vi "battery-reader-dialog.vi"() -> ()   [LabVIEW 2025]
uses:
  <vilib>/addons/_JKI Toolkits/State Machine/_JKI_lib_State_Machine.llb/Select State(s)_err__jki_lib_state_machine.vi
  <vilib>/addons/_JKI Toolkits/State Machine/_JKI_lib_State_Machine.llb/Periodic Trigger__ogtk__JKI-SM__jki_lib_state_machine.vi
panel:
  in  "Exit 2":bool
  in  "Exit":bool
  in  "Select":bool
  in  "Image selection":enum32{"Camera", "File input"}(tab)
  in  "Pict Ring":u16(ring)
  out "error out":errorcluster
  in  "error in":errorcluster
  in  "Camera ID":u8
  # "1. Select the camera ID and read the image."
  # "2. Use camera input, or select one of the predefined templates."
  # "3."
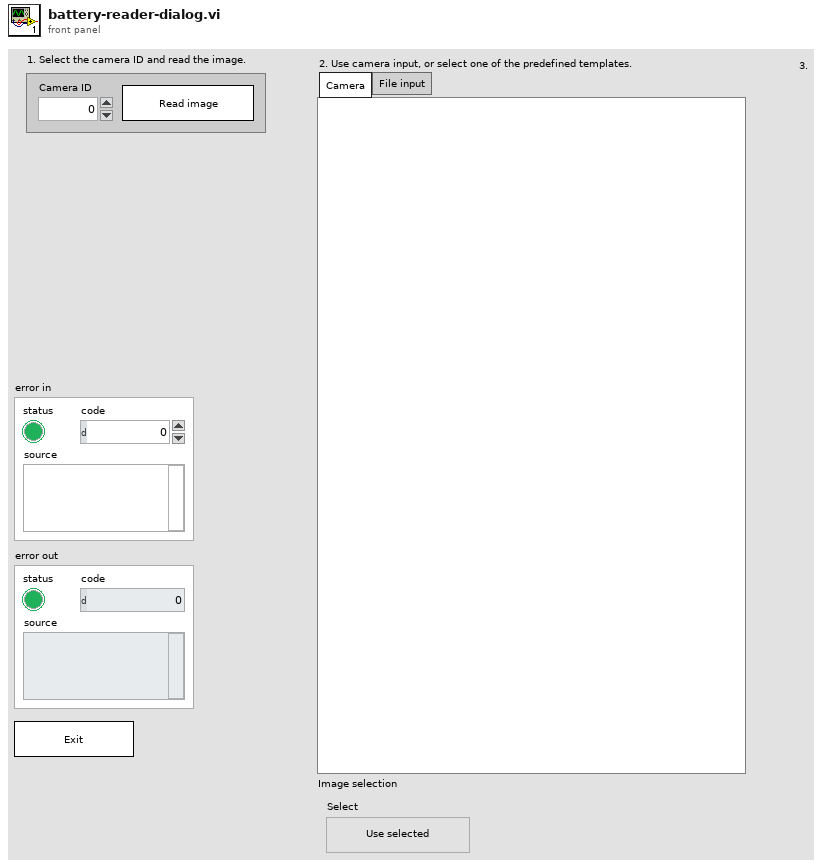
[diagram p1: front panel]
types:
  T1 = enum32{"Invalid", "Standard", "Closed", "Hidden", "Minimized", "Maximized"}
  T2 = enum32{"invalid app kind", "Development System", "Run Time System", "Student Edition", "Embedded LabVIEW", "Evaluation", "Custom"}
  T3 = cluster{"Core":cluster{"Current VI Reference":refnum<vi>, "Close Panel on Exit?":bool}, "Your Boolean data":bool, "Your string data":string}
  T4 = cluster{"Current VI Reference":refnum<vi>, "Close Panel on Exit?":bool}
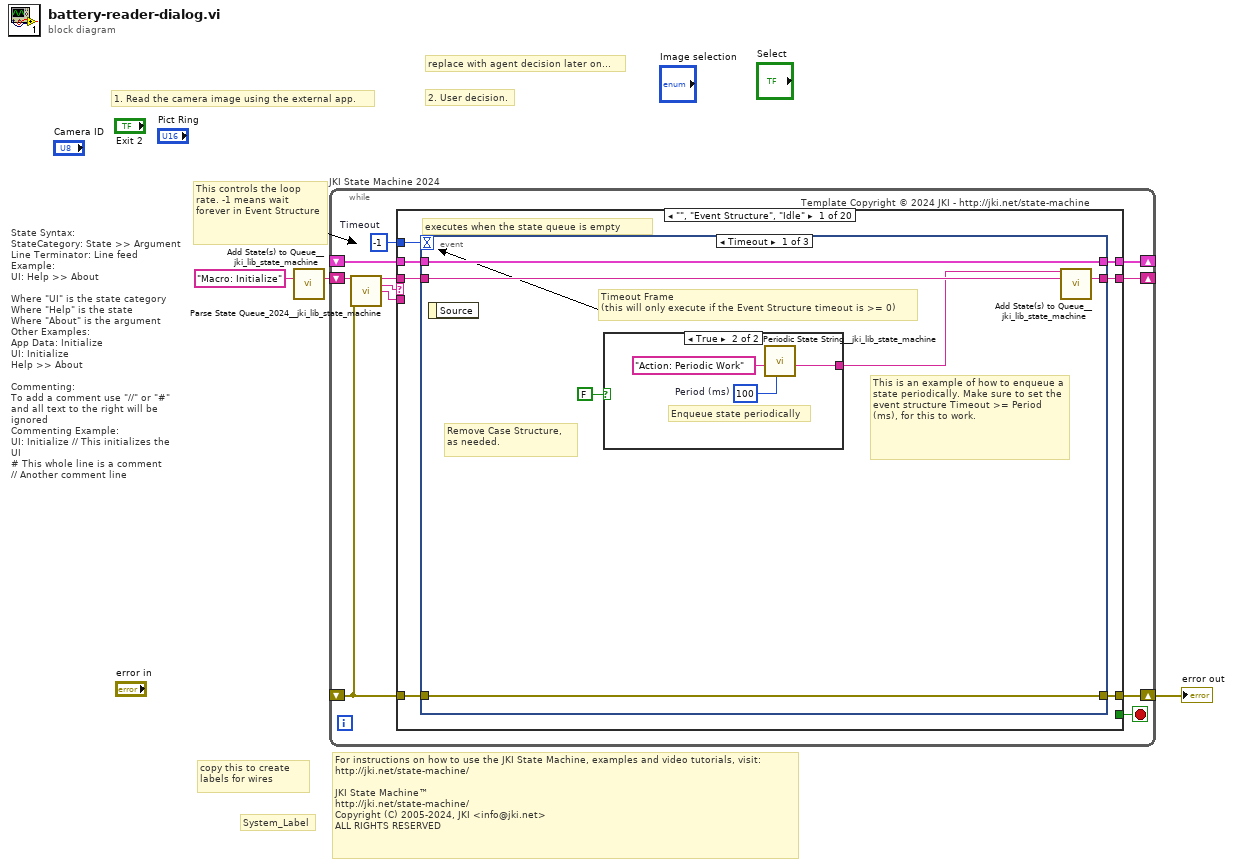
[diagram p0: block diagram]
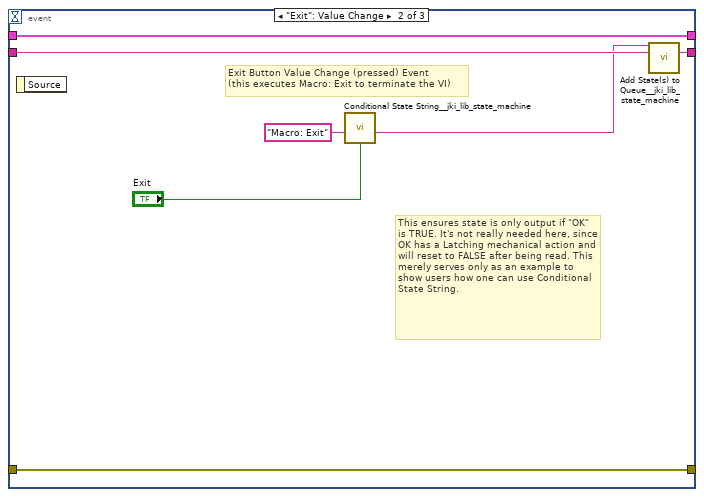
[diagram p3: hidden frame]
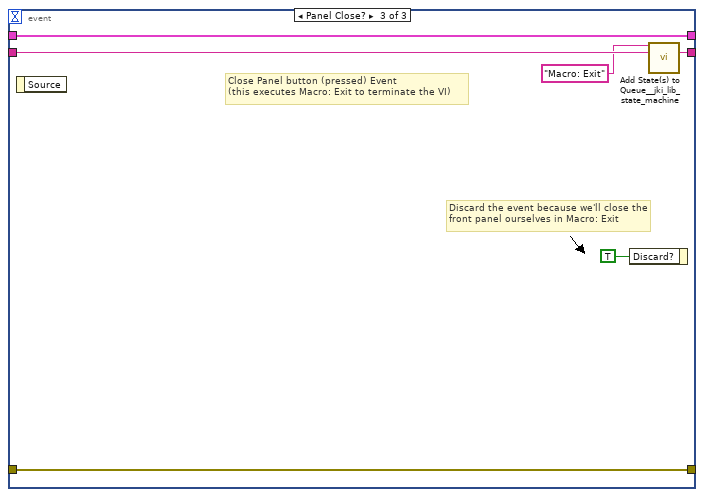
[diagram p4: hidden frame]
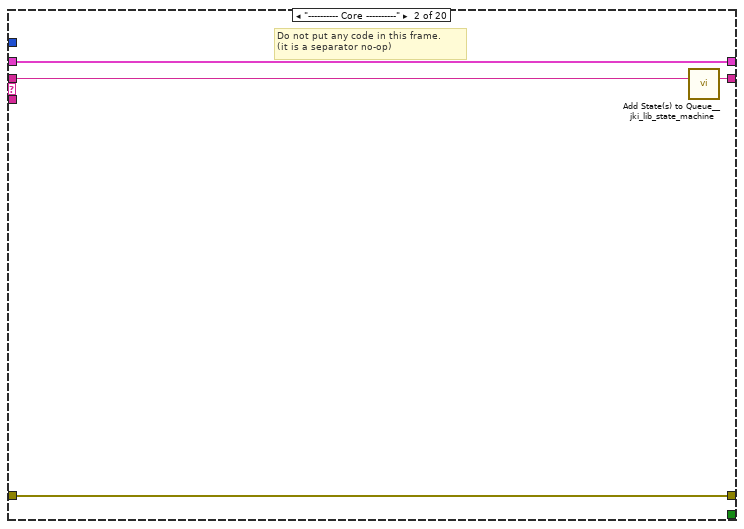
[diagram p5: hidden frame]
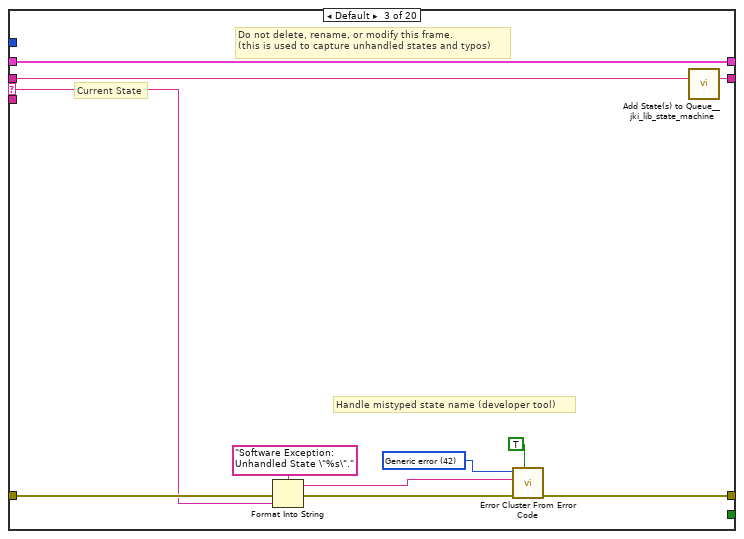
[diagram p6: hidden frame]
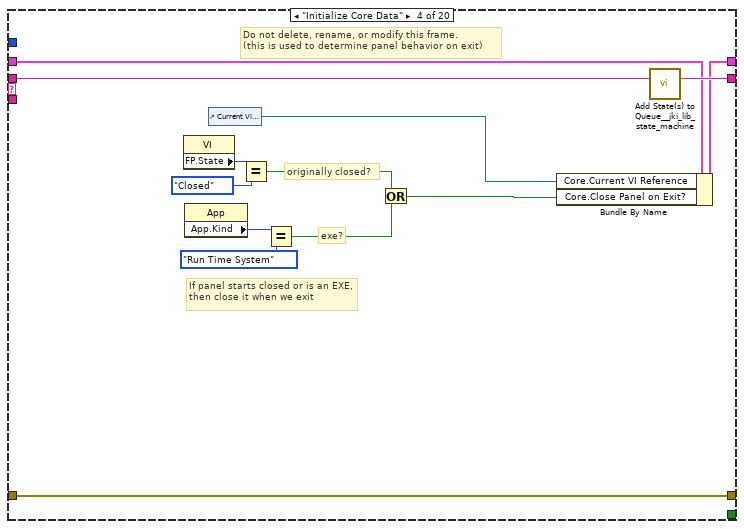
[diagram p7: hidden frame]
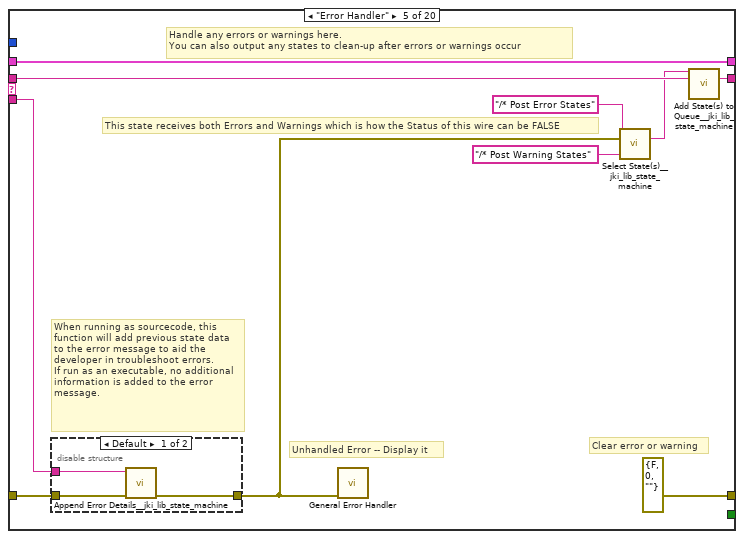
[diagram p8: hidden frame]
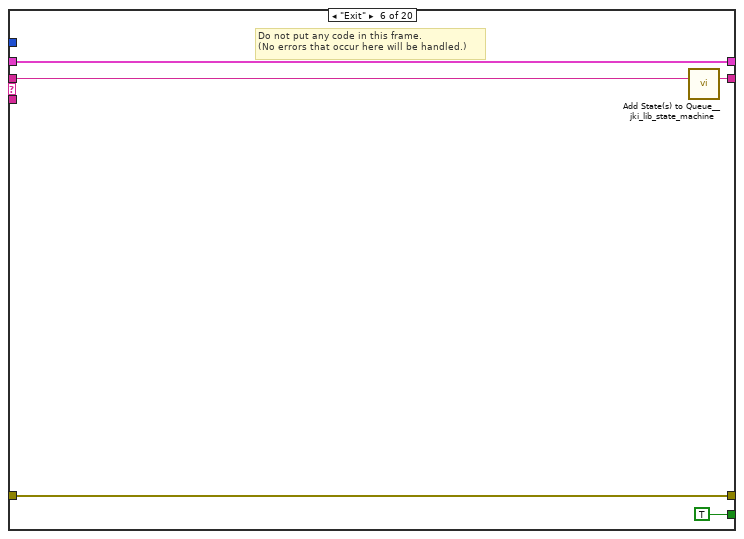
[diagram p10: hidden frame]
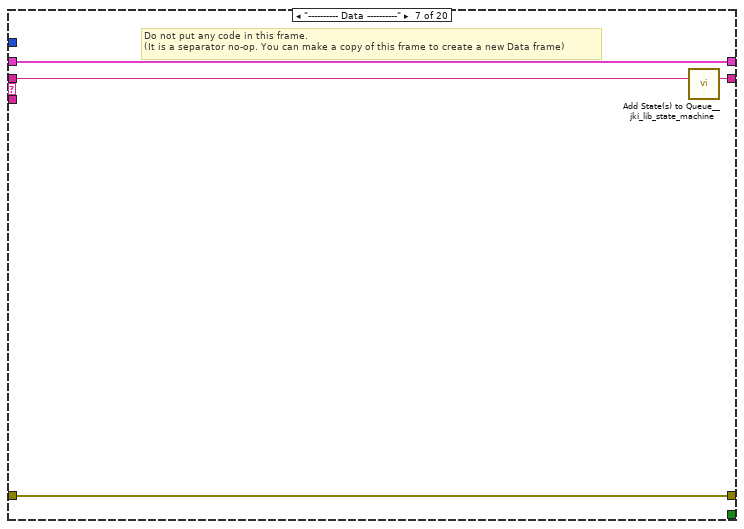
[diagram p11: hidden frame]
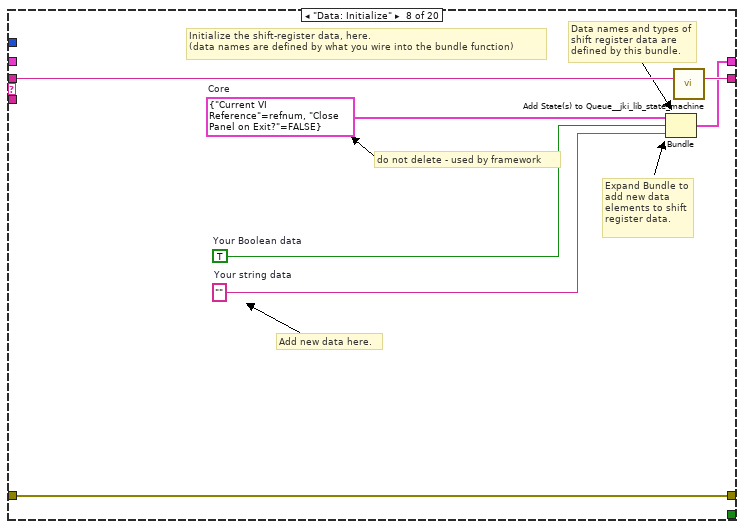
[diagram p12: hidden frame]
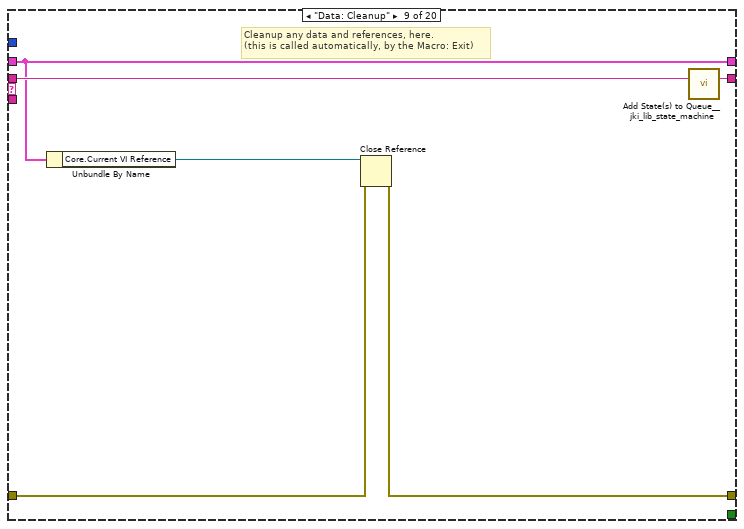
[diagram p13: hidden frame]
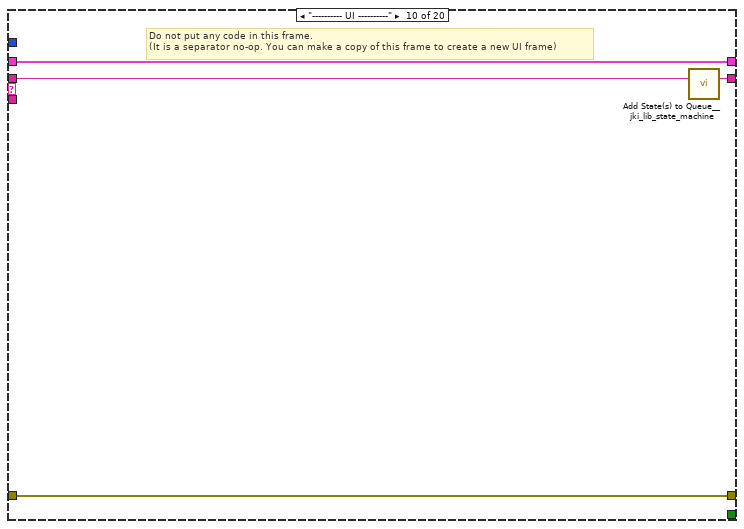
[diagram p14: hidden frame]
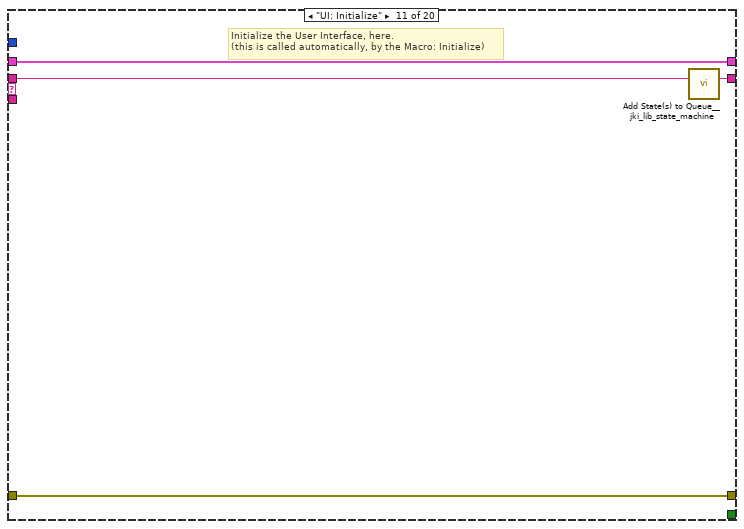
[diagram p15: hidden frame]
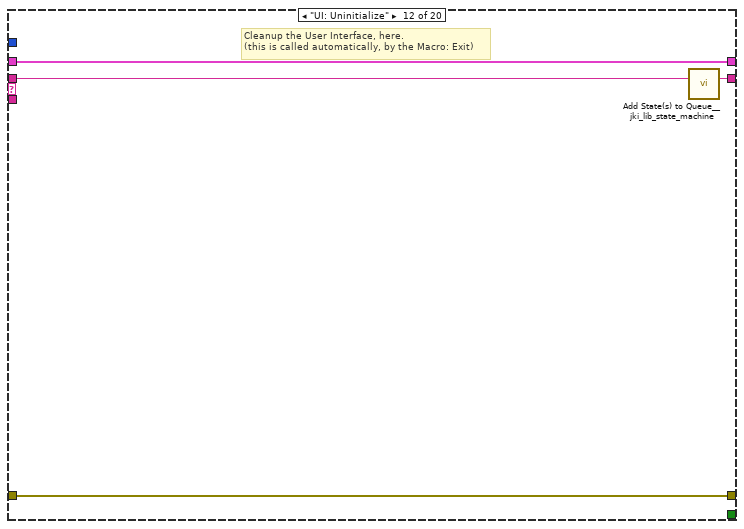
[diagram p16: hidden frame]
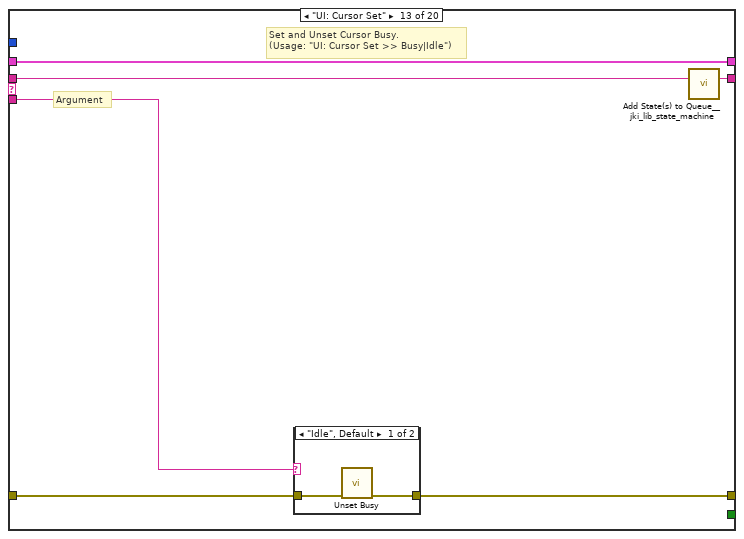
[diagram p17: hidden frame]
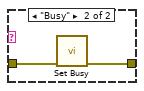
[diagram p18: hidden frame]
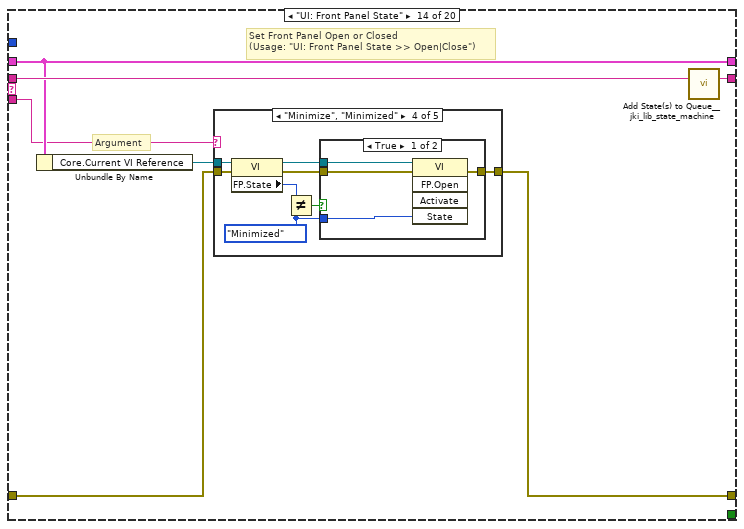
[diagram p19: hidden frame]
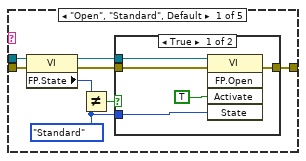
[diagram p20: hidden frame]
diagram:
  # "For instructions on how to use the JKI State Machine, examples and video tutorials, visit:\nhttp://jki.net/state-machine/\n\nJKI State Machine™\nhttp://jki.net/state-machine/\nCopyright (C) 2005-2024, JKI <info@jki.net>\nALL RIGHTS RESERVED"
  # "State Syntax:\nStateCategory: State >> Argument\nLine Terminator: Line feed\nExample:\nUI: Help >> About\n\nWhere \"UI\" is the state category\nWhere \"Help\" is the state\nWhere \"About\" is the argument\nOther Examples:\nApp Data: Initialize\nUI: Initialize\nHelp >> About\n\nCommenting:\nTo add a comment use \"//\" or \"#\" and all text to the right will be ignored\nCommenting Example:\nUI: Initialize // This initializes the UI\n# This whole line is a comment\n// Another comment line"
  # "copy this to create labels for wires"
  # "This controls the loop rate. -1 means wait forever in Event Structure"
  # "System_Label"
  # "replace with agent decision later on..."
  # "2. User decision."
  # "1. Read the camera image using the external app."
  n1 = call <vilib>:"Add State(s) to Queue__jki_lib_state_machine.vi"("State(s) in (\"\")"="Macro: Initialize") -> ("States Out"=w3:string)  [unwired: 14 in]
  n2 = while "JKI State Machine 2024" {
    shift-right: [w7] -> _
    shift-left: _ -> [w6]
    shift-right: [w10] -> w1
    shift-left: _ -> [w4]
    shift-right: [w9] -> _
    shift-left: w3 -> [w11]
    stop <- w8 stop-if-true
    w5 = -1  # Timeout
    # "Template Copyright © 2024 JKI - http://jki.net/state-machine"
    n3 = call <vilib>:"Parse State Queue_2024__jki_lib_state_machine.vi"("State Queue"=w11, "Error In (no error)"=w4) -> ("Remaining States"=w13:string, "Current State"=w14:string, "Arguments"=w12:string)  [unwired: 11 in]
    n4 = case shown="\"\", \"Event Structure\", \"Idle\"" w14 {
      selector: w14 -> [_ _ w48 _ _ _ _ _ _ _ _ _ _ _ _ _ _ _ _ _]
      tunnel: w13 -> [w21 w47 w52 w71 w81 w90 w94 w101 w107 w111 w115 w119 w125 w136 w205 w210 w219 w223 w227 w231]
      tunnel: w12 -> [_ _ _ _ w76 _ _ _ _ _ _ _ w120 w130 _ _ _ _ _ _]
      tunnel: w6 -> [w19 w44 w50 w64 w78 w88 w91 _ w102 w108 w113 w117 w123 w132 w202 w207 w217 w220 w224 w228]
      tunnel: [w18 w45 w54 w68 errorcluster {"status"=FALSE, "code"=0, "source"=""} ("error out") w87 w92 w98 w103 w109 w112 w116 w121 w133 w203 w208 w214 w221 w225 w229] -> w10
      tunnel: w4 -> [w15 w45 w53 w68 w77 w87 w92 w98 w104 w109 w112 w116 w122 w134 w203 w208 w214 w221 w225 w229]
      tunnel: [w20 w46 w51 w70 w80 w89 w93 w100 w106 w110 w114 w118 w124 w135 w204 w209 w218 w222 w226 w230] -> w9
      tunnel: [_ _ _ _ _ TRUE _ _ _ _ _ _ _ _ _ _ _ _ _ _] -> w8
      tunnel: [w17 w44 w50 w69 w78 w88 w91 w99 w102 w108 w113 w117 w123 w132 w202 w207 w217 w220 w224 w228] -> w7
      tunnel: w5 -> [w16 _ _ _ _ _ _ _ _ _ _ _ _ _ _ _ _ _ _ _]
      frame "", "Event Structure", "Idle" {
        # "executes when the state queue is empty"
        n5 = event shown="[0] Timeout" {
          selector: _ -> [_ _ _]
          dyn-events: _ -> [_ _ _]
          timeout: w16 -> [_ _ _]
          tunnel: w21 -> [w27 w37 w43]
          tunnel: [w26 w36 w42] -> w20
          tunnel: w19 -> [w24 w34 w40]
          tunnel: [w25 w35 w41] -> w18
          tunnel: w15 -> [w25 w35 w41]
          tunnel: [w24 w34 w40] -> w17
          event Timeout {
            # "Remove Case Structure, as needed."
            # "This is an example of how to enqueue a state periodically. Make sure to set the event structure Timeout >= Period (ms), for this to work."
            # "Timeout Frame\n(this will only execute if the Event Structure timeout is >= 0)"
            n6 = event-data() -> ()  [unwired: 1 in, 1 out]
            n7 = case shown="True" FALSE {
              tunnel: [_ w30] -> w23
              frame False {
              }
              frame True {
                w28 = u32 100  # Period (ms)
                # "Enqueue state periodically"
                n8 = call <vilib>:"Periodic State String__jki_lib_state_machine.vi"("Period (ms)"=w28, "State"="Action: Periodic Work") -> ("State Out"=w30:string)  [unwired: 9 in]
              }
            }
            n9 = call <vilib>:"Add State(s) to Queue__jki_lib_state_machine.vi"("State(s) in Front (\"\")"=w23, "State(s) in (\"\")"=w27) -> ("States Out"=w26:string)  [unwired: 13 in]
          }
          event "Exit": Value Change {
            # "This ensures state is only output if \"OK\" is TRUE. It's not really needed here, since OK has a Latching mechanical action and will reset to FALSE after being read. This merely serves only as an example to show users how one can use Conditional State String."
            # "Exit Button Value Change (pressed) Event\n(this executes Macro: Exit to terminate the VI)"
            n10 = event-data() -> ()  [unwired: 1 in, 1 out]
            n11 = call <vilib>:"Conditional State String__jki_lib_state_machine.vi"("Do State(s)?"="Exit", "State"="Macro: Exit") -> ("State Out"=w31:string)  [unwired: 7 in]
            n12 = call <vilib>:"Add State(s) to Queue__jki_lib_state_machine.vi"("State(s) in Front (\"\")"=w31, "State(s) in (\"\")"=w37) -> ("States Out"=w36:string)  [unwired: 13 in]
          }
          event Panel Close? {
            # "Discard the event because we'll close the front panel ourselves in Macro: Exit"
            # "Close Panel button (pressed) Event\n(this executes Macro: Exit to terminate the VI)"
            n13 = event-data() -> ()  [unwired: 1 in, 1 out]
            n14 = event-data("Discard?"=TRUE) -> ()  [unwired: 1 in, 1 out]
            n15 = call <vilib>:"Add State(s) to Queue__jki_lib_state_machine.vi"("State(s) in Front (\"\")"="Macro: Exit", "State(s) in (\"\")"=w43) -> ("States Out"=w42:string)  [unwired: 13 in]
          }
        }
      }
      frame "---------- Core ----------" {
        # "Do not put any code in this frame.\n(it is a separator no-op)"
        n16 = call <vilib>:"Add State(s) to Queue__jki_lib_state_machine.vi"("State(s) in (\"\")"=w47) -> ("States Out"=w46:string)  [unwired: 14 in]
      }
      frame Default {
        w57 = 42 items=["No error", "Argument error", "Memory is full", "Out of zone", "End of file", "File already open", "Generic file I/O error", "File not found", "File permission error", "Disk is full", "Duplicate path", "Too many files open", "System feature not enabled", "Resource file not found", "Cannot add resource", "Resource not found", "Image not found", "Image memory error", "Pen does not exist", "Config type invalid", "Config token not found", "Config parse error", "Config memory error", "Bad external code format", "Bad external code offset", "External code not present", "Null window", "Destroy window error", "Null menu", "Print aborted", "Bad print record", "Print driver error", "Windows error during printing", "Memory error during printing", "Print dialog error", "Generic print error", "Invalid device refnum", "Device not found", "Device parameter error", "Device unit error", "Cannot open device", "Device call aborted", "Generic error", "Cancelled by user", "Object ID too low", "Object ID too high", "Object not in heap", "Unknown heap", "Unknown object (invalid DefProc)", "Unknown object (DefProc not in table)", "Message out of range", "Invalid (null) method", "Unknown message", "Manager call not supported", "Bad address", "Network operation in progress", "Network operation timed out", "Connection is busy", "Network attribute not supported", "Network error", "Address in use", "System out of memory", "Connection aborted", "Connection refused", "Not connected", "Already connected", "Connection closed", "Initialization error (interapplication manager)", "Bad occurrence", "Wait on unbound occurrence handler", "Occurrence queue overflow", "Datalog type conflict", "Unused", "Unrecognized type (interapplication manager)", "Memory corrupt", "Failed to make temporary DLL", "Old CIN version", "Drag socket not found", "Failed to load drop-object", "Failed to register OLE object", "Failed to release OLE object", "Format specifier type mismatch", "Unknown format specifier", "Too few format specifiers", "Too many format specifiers", "Scan failed", "Newer CIN version", "Error converting to variant", "Runtime menu error", "Password tampered", "Variant attribute not found", "Incompatible variant data type", "Event data is not available", "Event Store is not present", "Occurrence is not found", "Event Queue is not created", "Event info is not available", "Refnum passed is NULL", "Error retrieving Class GUID", "Error retrieving CoClass GUID", "Error retrieving TypeLib GUID.", "Bad built application magic bytes.", "Specific driver is different from the specific driver associated with the Logical Name.", "There is no session opened to the class driver.", "Max Error", "MAX - Error with config objects", "MAX - Error loading configuration", "MAX - Group not supported"]
        # "Current State"
        # "Do not delete, rename, or modify this frame.\n(this is used to capture unhandled states and typos)"
        # "Handle mistyped state name (developer tool)"
        n17 = Format Into String(format string="Software Exception: Unhandled State \"%s\"." ("message"), error in=w53, w48) -> (resulting string=w56:string, error out=w55:errorcluster)  [unwired: 1 in]
        n18 = call <vilib>:"Error Cluster From Error Code.vi"("show call chain? (False)"=TRUE, "error in (no error)"=w55, "error message (\"\")"=w56, "error code (0)"=w57) -> ("error out"=w54:errorcluster)  [unwired: 5 in]
        n19 = call <vilib>:"Add State(s) to Queue__jki_lib_state_machine.vi"("State(s) in (\"\")"=w52) -> ("States Out"=w51:string)  [unwired: 14 in]
      }
      frame "Initialize Core Data" {
        # "Do not delete, rename, or modify this frame.\n(this is used to determine panel behavior on exit)"
        # "originally closed?"
        # "exe?"
        # "If panel starts closed or is an EXE, then close it when we exit"
        n20 = property class="VI"() -> ("FP.State"=w61:T1)  [unwired: 2 in, 2 out]
        n21 = property class="App"() -> ("App.Kind"=w67:T2)  [unwired: 2 in, 2 out]
        n22 = control-ref of="Current VI Reference"() -> (w62:refnum<vi>)
        n23 = Equal?(x=w61, y=T1."Closed" ("Front Panel Window:State")) -> (x = y?=w59:bool)
        n24 = Equal?(x=w67, y=T2."Run Time System" ("Application:Kind")) -> (x = y?=w65:bool)
        n25 = Or(x=w59, y=w65) -> (x .or. y?=w63:bool)
        n26 = Bundle By Name(cluster=w64, "Core.Current VI Reference"=w62, "Core.Close Panel on Exit?"=w63) -> (w69:T3)
        n27 = call <vilib>:"Add State(s) to Queue__jki_lib_state_machine.vi"("State(s) in (\"\")"=w71) -> ("States Out"=w70:string)  [unwired: 14 in]
      }
      frame "Error Handler" {
        # "When running as sourcecode, this function will add previous state data to the error message to aid the developer in troubleshoot errors.\nIf run as an executable, no additional information is added to the error message."
        # "This state receives both Errors and Warnings which is how the Status of this wire can be FALSE"
        # "Unhandled Error -- Display it"
        # "Handle any errors or warnings here.\nYou can also output any states to clean-up after errors or warnings occur"
        # "Clear error or warning"
        n28 = disable-structure shown="Default" {
          disable-tunnel: w77 -> [w84 w85]
          disable-tunnel: w76 -> [w83 _]
          disable-tunnel: [w82 w85] -> w75
          frame condition #0 (active) {
            n29 = call <vilib>:"Append Error Details__jki_lib_state_machine.vi"("error in (no error)"=w84, "Previous State and Argument(s)"=w83) -> ("error out"=w82:errorcluster)  [unwired: 9 in]
          }
          frame condition #1 {
          }
        }
        n30 = call <vilib>:"General Error Handler.vi"("error in (no error)"=w75) -> ()  [unwired: 10 in, 5 out]
        n31 = call-poly <vilib>:"Select State(s)__jki_lib_state_machine.vi"("State(s) if True (\"\")"="/* Post Error States", "Select"=w75, "State(s) if False (\"\")"="/* Post Warning States") -> ("States Out"=w73:string)  [unwired: 12 in]
        n32 = call <vilib>:"Add State(s) to Queue__jki_lib_state_machine.vi"("State(s) in Front (\"\")"=w73, "State(s) in (\"\")"=w81) -> ("States Out"=w80:string)  [unwired: 13 in]
      }
      frame "Exit" {
        # "Do not put any code in this frame.\n(No errors that occur here will be handled.)"
        n33 = call <vilib>:"Add State(s) to Queue__jki_lib_state_machine.vi"("State(s) in (\"\")"=w90) -> ("States Out"=w89:string)  [unwired: 14 in]
      }
      frame "---------- Data ----------" {
        # "Do not put any code in this frame.\n(It is a separator no-op. You can make a copy of this frame to create a new Data frame)"
        n34 = call <vilib>:"Add State(s) to Queue__jki_lib_state_machine.vi"("State(s) in (\"\")"=w94) -> ("States Out"=w93:string)  [unwired: 14 in]
      }
      frame "Data: Initialize" {
        w95 = T4 {"Current VI Reference"=refnum, "Close Panel on Exit?"=FALSE}  # Core
        w97 = TRUE  # Your Boolean data
        w96 = ""  # Your string data
        # "do not delete - used by framework"
        # "Expand Bundle to add new data elements to shift register data."
        # "Add new data here."
        # "Data names and types of shift register data are defined by this bundle."
        # "Initialize the shift-register data, here.\n(data names are defined by what you wire into the bundle function)"
        n35 = Bundle("Core"=w95, "Your Boolean data"=w97, "Your string data"=w96) -> (w99:T3)  [unwired: 1 in]
        n36 = call <vilib>:"Add State(s) to Queue__jki_lib_state_machine.vi"("State(s) in (\"\")"=w101) -> ("States Out"=w100:string)  [unwired: 14 in]
      }
      frame "Data: Cleanup" {
        # "Cleanup any data and references, here.\n(this is called automatically, by the Macro: Exit)"
        n37 = Unbundle By Name(w102) -> ("Core.Current VI Reference"=w105:refnum<vi>)
        n38 = Close Reference(reference=w105, error in (no error)=w104) -> (error out=w103:errorcluster)
        n39 = call <vilib>:"Add State(s) to Queue__jki_lib_state_machine.vi"("State(s) in (\"\")"=w107) -> ("States Out"=w106:string)  [unwired: 14 in]
      }
      frame "---------- UI ----------" {
        # "Do not put any code in this frame.\n(It is a separator no-op. You can make a copy of this frame to create a new UI frame)"
        n40 = call <vilib>:"Add State(s) to Queue__jki_lib_state_machine.vi"("State(s) in (\"\")"=w111) -> ("States Out"=w110:string)  [unwired: 14 in]
      }
      frame "UI: Initialize" {
        # "Initialize the User Interface, here.\n(this is called automatically, by the Macro: Initialize)"
        n41 = call <vilib>:"Add State(s) to Queue__jki_lib_state_machine.vi"("State(s) in (\"\")"=w115) -> ("States Out"=w114:string)  [unwired: 14 in]
      }
      frame "UI: Uninitialize" {
        # "Cleanup the User Interface, here.\n(this is called automatically, by the Macro: Exit)"
        n42 = call <vilib>:"Add State(s) to Queue__jki_lib_state_machine.vi"("State(s) in (\"\")"=w119) -> ("States Out"=w118:string)  [unwired: 14 in]
      }
      frame "UI: Cursor Set" {
        # "Argument"
        # "Set and Unset Cursor Busy.\n(Usage: \"UI: Cursor Set >> Busy|Idle\")"
        n43 = case shown="\"Idle\", Default" w120 {
          tunnel: w122 -> [w127 w129]
          tunnel: [w126 w128] -> w121
          frame "Idle", Default {
            n44 = call <vilib>:"Unset Busy.vi"("error in (no error)"=w127) -> ("error out"=w126:errorcluster)  [unwired: 10 in]
          }
          frame "Busy" {
            n45 = call <vilib>:"Set Busy.vi"("error in (no error)"=w129) -> ("error out"=w128:errorcluster)  [unwired: 9 in, 1 out]
          }
        }
        n46 = call <vilib>:"Add State(s) to Queue__jki_lib_state_machine.vi"("State(s) in (\"\")"=w125) -> ("States Out"=w124:string)  [unwired: 14 in]
      }
      frame "UI: Front Panel State" {
        # "Argument"
        # "Set Front Panel Open or Closed\n(Usage: \"UI: Front Panel State >> Open|Close\")"
        n47 = Unbundle By Name(w132) -> ("Core.Current VI Reference"=w131:refnum<vi>)
        n48 = case shown="\"Minimize\", \"Minimized\"" w130 {
          tunnel: w134 -> [w142 w157 w168 w181 w194]
          tunnel: [w144 w158 w170 w183 w196] -> w133
          tunnel: w131 -> [w143 w155 w169 w182 w195]
          frame "Open", "Standard", Default {
            w137 = T1."Standard" ("State")
            n49 = property class="VI"(reference=w143, error in=w142) -> (reference out=w140:refnum<vi>, error out=w141:errorcluster, "FP.State"=w139:T1)
            n50 = Not Equal?(x=w139, y=w137) -> (x != y?=w138:bool)
            n51 = case shown="True" w138 {
              tunnel: [w148 w150] -> w144
              tunnel: w141 -> [w147 w150]
              tunnel: w140 -> [w146 _]
              tunnel: w137 -> [w145 _]
              frame True {
                n52 = invoke class="VI" method="FP.Open"(reference=w146, error in=w147, "Activate"=TRUE, "State"=w145) -> (error out=w148:errorcluster)  [unwired: 1 in, 4 out]
              }
              frame False {
              }
            }
          }
          frame "Close", "Closed" {
            n53 = property class="VI"(reference=w155, error in=w157) -> (reference out=w154:refnum<vi>, error out=w156:errorcluster, "FP.State"=w152:T1)
            n54 = Not Equal?(x=w152, y=T1."Closed" ("Front Panel Window:State")) -> (x != y?=w151:bool)
            n55 = case shown="True" w151 {
              tunnel: [w159 w162] -> w158
              tunnel: w156 -> [w159 w161]
              tunnel: w154 -> [_ w160]
              frame False {
              }
              frame True {
                n56 = invoke class="VI" method="FP.Close"(reference=w160, error in=w161) -> (error out=w162:errorcluster)  [unwired: 1 in, 2 out]
              }
            }
          }
          frame "Hidden", "Hide" {
            w163 = T1."Hidden" ("State")
            n57 = property class="VI"(reference=w169, error in=w168) -> (reference out=w166:refnum<vi>, error out=w167:errorcluster, "FP.State"=w165:T1)
            n58 = Not Equal?(x=w165, y=w163) -> (x != y?=w164:bool)
            n59 = case shown="True" w164 {
              tunnel: [w174 w175] -> w170
              tunnel: w167 -> [w173 w175]
              tunnel: w166 -> [w172 _]
              tunnel: w163 -> [w171 _]
              frame True {
                n60 = invoke class="VI" method="FP.Open"(reference=w172, error in=w173, "State"=w171) -> (error out=w174:errorcluster)  [unwired: 2 in, 4 out]
              }
              frame False {
              }
            }
          }
          frame "Minimize", "Minimized" {
            w176 = T1."Minimized" ("State")
            n61 = property class="VI"(reference=w182, error in=w181) -> (reference out=w179:refnum<vi>, error out=w180:errorcluster, "FP.State"=w178:T1)
            n62 = Not Equal?(x=w178, y=w176) -> (x != y?=w177:bool)
            n63 = case shown="True" w177 {
              tunnel: [w187 w188] -> w183
              tunnel: w180 -> [w186 w188]
              tunnel: w179 -> [w185 _]
              tunnel: w176 -> [w184 _]
              frame True {
                n64 = invoke class="VI" method="FP.Open"(reference=w185, error in=w186, "State"=w184) -> (error out=w187:errorcluster)  [unwired: 2 in, 4 out]
              }
              frame False {
              }
            }
          }
          frame "Maximize", "Maximized" {
            w189 = T1."Maximized" ("State")
            n65 = property class="VI"(reference=w195, error in=w194) -> (reference out=w192:refnum<vi>, error out=w193:errorcluster, "FP.State"=w191:T1)
            n66 = Not Equal?(x=w191, y=w189) -> (x != y?=w190:bool)
            n67 = case shown="True" w190 {
              tunnel: [w200 w201] -> w196
              tunnel: w193 -> [w199 w201]
              tunnel: w192 -> [w198 _]
              tunnel: w189 -> [w197 _]
              frame True {
                n68 = invoke class="VI" method="FP.Open"(reference=w198, error in=w199, "State"=w197) -> (error out=w200:errorcluster)  [unwired: 2 in, 4 out]
              }
              frame False {
              }
            }
          }
        }
        n69 = call <vilib>:"Add State(s) to Queue__jki_lib_state_machine.vi"("State(s) in (\"\")"=w136) -> ("States Out"=w135:string)  [unwired: 14 in]
      }
      frame "---------- Macro ----------" {
        # "Do not put any code in this frame.\n(It is a separator no-op. You can make a copy of this frame to create a new Macro frame)"
        n70 = call <vilib>:"Add State(s) to Queue__jki_lib_state_machine.vi"("State(s) in (\"\")"=w205) -> ("States Out"=w204:string)  [unwired: 14 in]
      }
      frame "Macro: Initialize" {
        w206 = "Data: Initialize\nInitialize Core Data\nUI: Initialize\nUI: Front Panel State >> Open"  # Data: Initialize Initialize Core Data UI: Initialize UI: Front Panel State >> Open
        # "Initialization Macro\n(This is called once, when the VI starts)"
        n71 = call <vilib>:"Add State(s) to Queue__jki_lib_state_machine.vi"("State(s) in Front (\"\")"=w206, "State(s) in (\"\")"=w210) -> ("States Out"=w209:string)  [unwired: 13 in]
      }
      frame "Macro: Exit" {
        # "Exit Macro\n(This is called once, when the VI exits)"
        n72 = Unbundle By Name(w217) -> ("Core.Close Panel on Exit?"=w212:bool)
        n73 = call <vilib>:"Conditional State String__jki_lib_state_machine.vi"("Do State(s)?"=w212, "State"="UI: Front Panel State >> Close") -> ("State Out"=w211:string)  [unwired: 7 in]
        n74 = call <vilib>:"Add State(s) to Queue__jki_lib_state_machine.vi"("State(s) in (\"\")"=w211, "State(s) at Back (\"\")"="UI: Uninitialize\nData: Cleanup\nExit") -> ("States Out"=w215:string)  [unwired: 13 in]
        n75 = call <vilib>:"Add State(s) to Queue__jki_lib_state_machine.vi"("State(s) in Front (\"\")"=w215, "State(s) in (\"\")"=w219) -> ("States Out"=w218:string)  [unwired: 13 in]
      }
      frame "---------- New Category ----------" {
        # "Template Separator\n(You can make a copy of, or modify, this frame)"
        n76 = call <vilib>:"Add State(s) to Queue__jki_lib_state_machine.vi"("State(s) in (\"\")"=w223) -> ("States Out"=w222:string)  [unwired: 14 in]
      }
      frame "New Category: 1" {
        # "Your code here.\n(You can make a copy of, or modify, this frame)"
        n77 = call <vilib>:"Add State(s) to Queue__jki_lib_state_machine.vi"("State(s) in (\"\")"=w227) -> ("States Out"=w226:string)  [unwired: 14 in]
      }
      frame "New Category: 2" {
        # "Your code here.\n(You can make a copy of, or modify, this frame)"
        n78 = call <vilib>:"Add State(s) to Queue__jki_lib_state_machine.vi"("State(s) in (\"\")"=w231) -> ("States Out"=w230:string)  [unwired: 14 in]
      }
    }
  }
  "error out" <- w1
